vi "HEWH Mixing Valve.vi"(8 "Error In":errorcluster, 9 "Disable ERD (Main)":bool, 10 "ERD Data Out":T4[](array[typedef]) {"ERD Number" format="%.0x"}, 11 "ERD Data":T1 {"ERD Therm Data"."EEV Possition" format="%0.0f"; "ERD Therm Data"."T6" format="%.1f"; "ERD Therm Data"."T2" format="%.1f"; "ERD Therm Data"."T3a" format="%.1f"; "ERD Therm Data"."T3b" format="%.1f"; "ERD Therm Data"."T4" format="%.1f"; "ERD Therm Data"."T5" format="%.1f"; "ERD Therm Data"."Current" format="%.1f"}) -> (0 "Error Out":errorcluster, 3 "ERD Data Out":T1 {"ERD Therm Data"."EEV Possition" format="%0.0f"; "ERD Therm Data"."T6" format="%.1f"; "ERD Therm Data"."T2" format="%.1f"; "ERD Therm Data"."T3a" format="%.1f"; "ERD Therm Data"."T3b" format="%.1f"; "ERD Therm Data"."T4" format="%.1f"; "ERD Therm Data"."T5" format="%.1f"; "ERD Therm Data"."Current" format="%.1f"})   [LabVIEW 2016]
uses:
  type defs/ERD Read Data Out.ctl
  type defs/HEWH ERD Data.ctl
  type defs/HEWH Faults.ctl
  type defs/HEWH Mixing Valve.ctl
  library/GEA2_Toolkit.lvlib
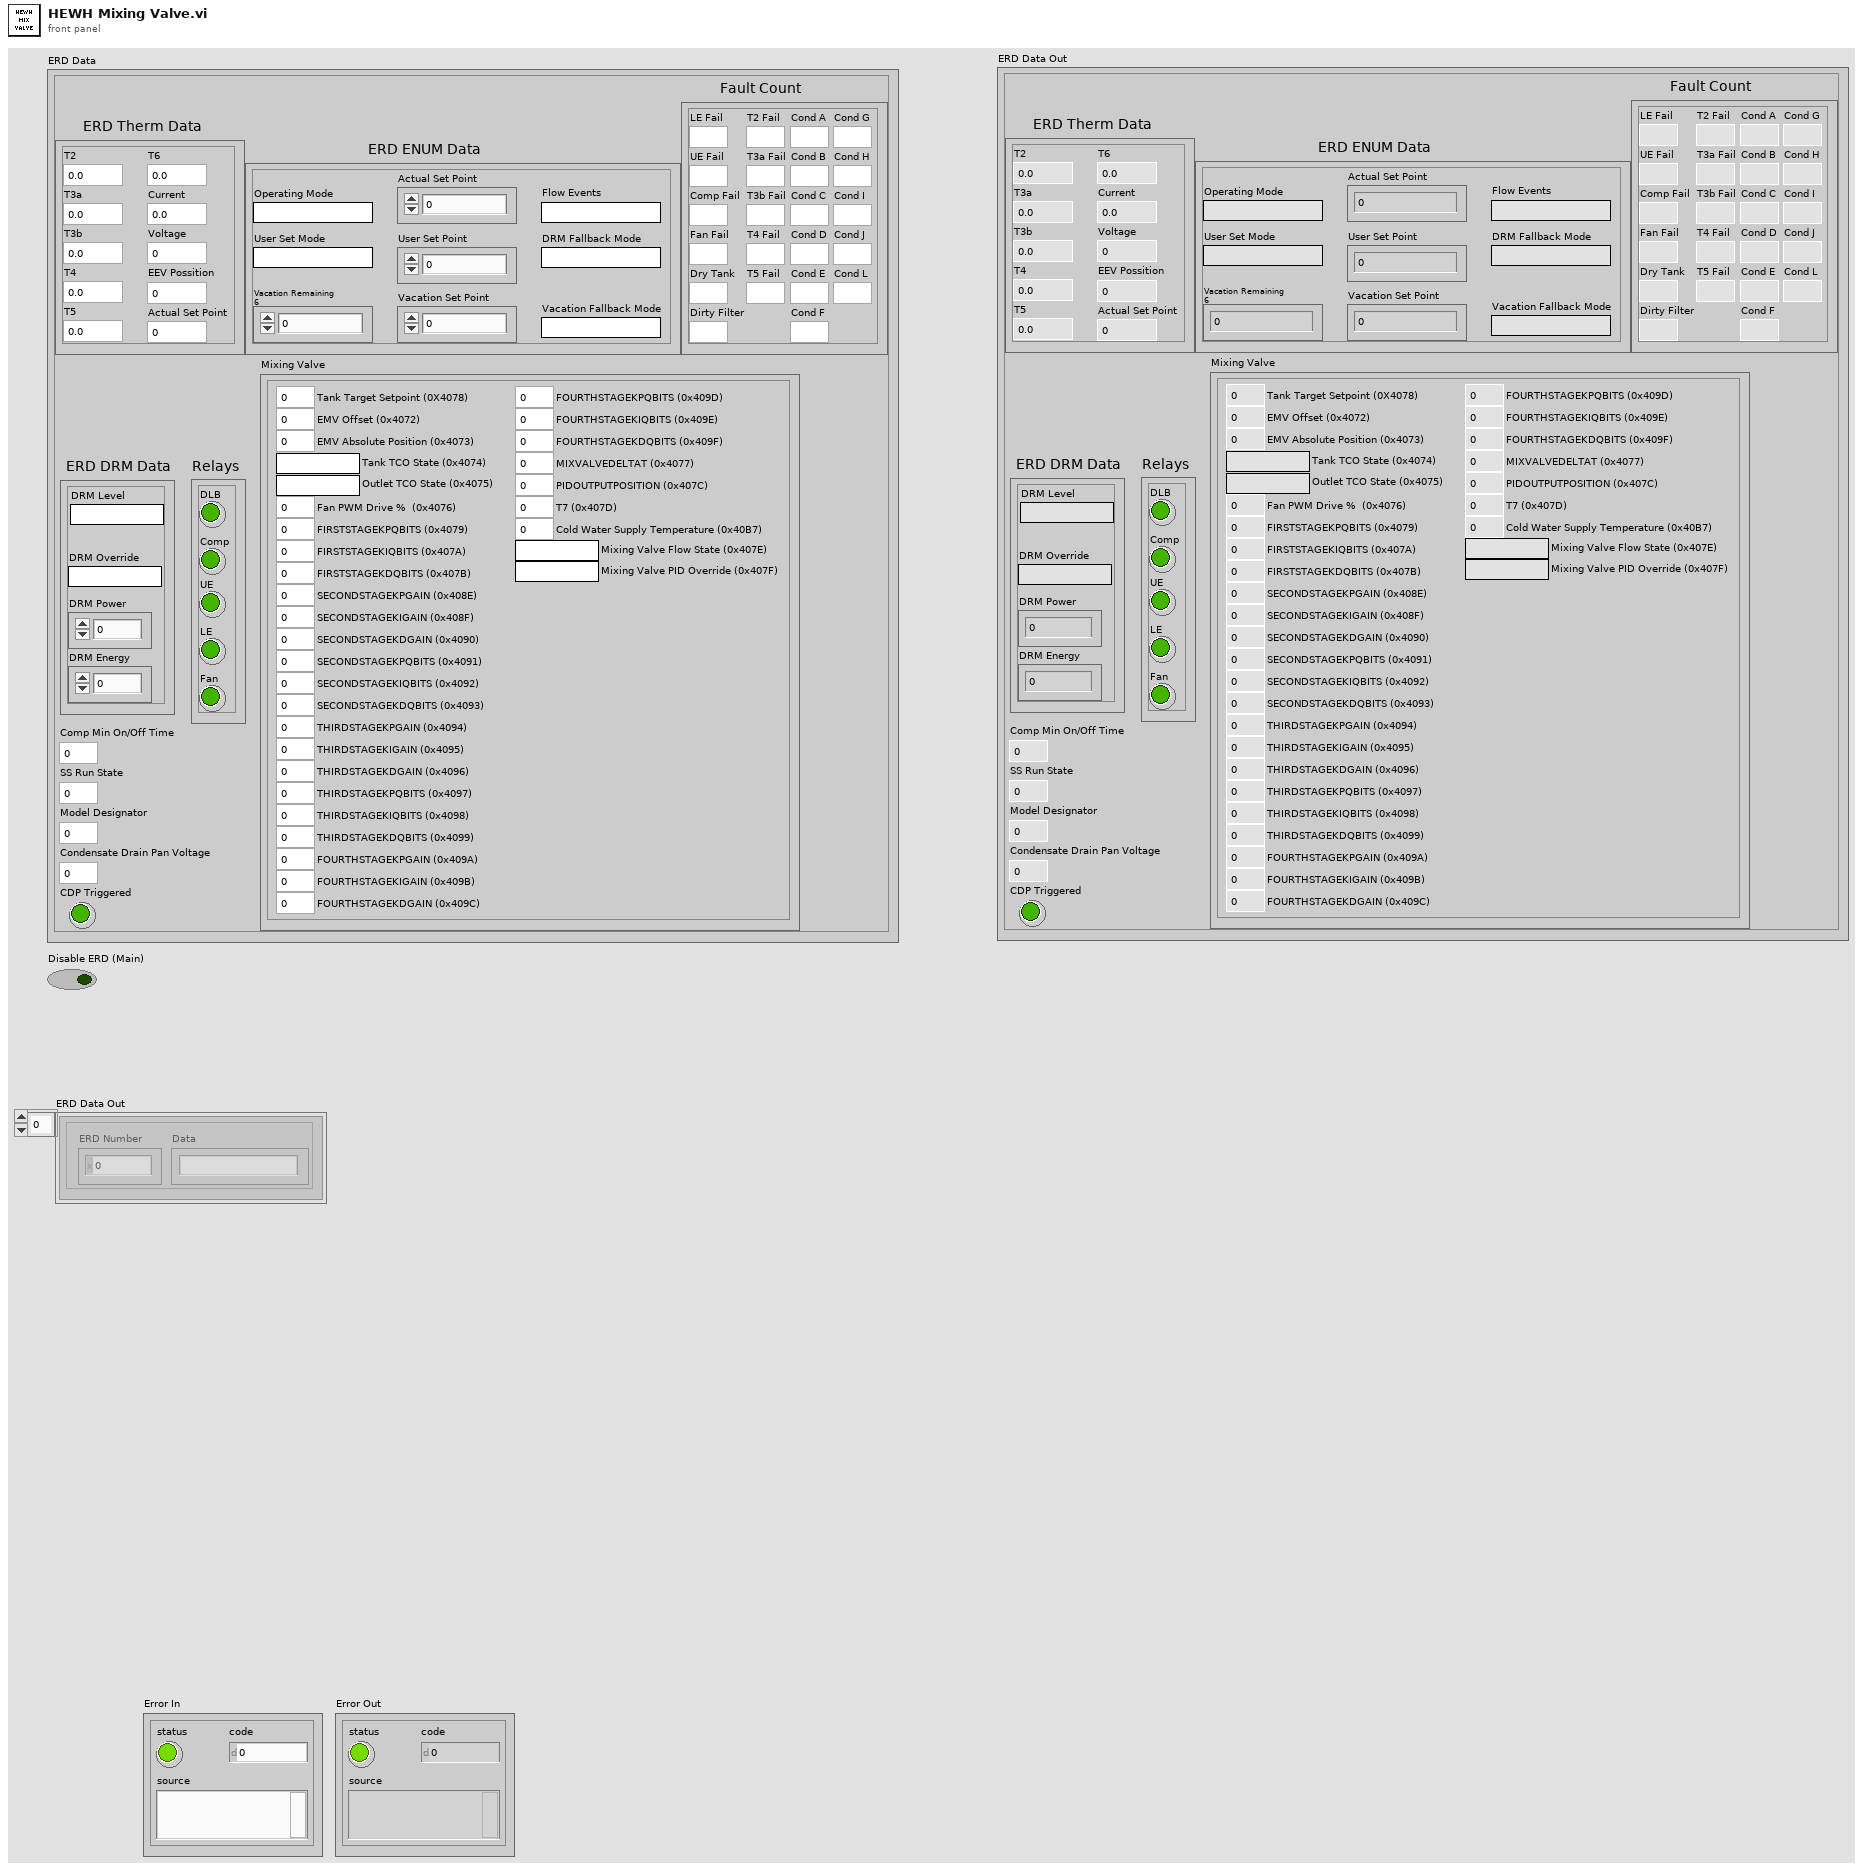
[diagram p1: front panel]
types:
  T1 = typedef "HEWH ERD Data.ctl" = cluster{"ERD Therm Data":cluster{"T2":dbl, "T3a":dbl, "T3b":dbl, "T4":dbl, "T5":dbl, "T6":dbl, "Current":dbl, "Voltage":dbl, "EEV Possition":dbl, "Actual Set Point":dbl}, "ERD ENUM Data":cluster{"Actual Set Point":dbl, "Flow Events":string, "User Set Mode":string, "Operating Mode":string, "DRM Fallback Mode":string, "Vacation Fallback Mode":string, "User Set Point":dbl, "Vacation Set Point":dbl, "Vacation Remaining\n6":dbl}, "ERD DRM Data":cluster{"DRM Level":string, "DRM Override":string, "DRM Power":dbl, "DRM Energy":dbl}, "Fault Count":T2, "Relays":cluster{"DLB":bool, "Comp":bool, "UE":bool, "LE":bool, "Fan":bool}, "Comp Min On/Off Time":u16, "SS Run State":u16, "Condensate Drain Pan Voltage":u16, "CDP Triggered":bool, "Model Designator":u8, "Mixing Valve":T3}
  T2 = typedef "HEWH Faults.ctl" = cluster{"LE Fail":u32, "UE Fail":u32, "Comp Fail":u32, "T2 Fail":u32, "T3a Fail":u32, "T3b Fail":u32, "T4 Fail":u32, "T5 Fail":u32, "Cond A":u32, "Cond B":u32, "Cond C":u32, "Cond D":u32, "Cond E":u32, "Cond F":u32, "Cond G":u32, "Cond H":u32, "Cond I":u32, "Cond J":u32, "Cond L":u32, "Fan Fail":u32, "Dirty Filter":u32, "Dry Tank":u32}
  T3 = typedef "HEWH Mixing Valve.ctl" = cluster{"Tank Target Setpoint (0X4078)":dbl, "EMV Offset (0x4072)":dbl, "EMV Absolute Position (0x4073)":dbl, "Tank TCO State (0x4074)":string, "Outlet TCO State (0x4075)":string, "Fan PWM Drive %  (0x4076)":dbl, "FIRSTSTAGEKPQBITS (0x4079)":dbl, "FIRSTSTAGEKIQBITS (0x407A)":dbl, "FIRSTSTAGEKDQBITS (0x407B)":dbl, "SECONDSTAGEKPGAIN (0x408E)":dbl, "SECONDSTAGEKIGAIN (0x408F)":dbl, "SECONDSTAGEKDGAIN (0x4090)":dbl, "SECONDSTAGEKPQBITS (0x4091)":dbl, "SECONDSTAGEKIQBITS (0x4092)":dbl, "SECONDSTAGEKDQBITS (0x4093)":dbl, "THIRDSTAGEKPGAIN (0x4094)":dbl, "THIRDSTAGEKIGAIN (0x4095)":dbl, "THIRDSTAGEKDGAIN (0x4096)":dbl, "THIRDSTAGEKPQBITS (0x4097)":dbl, "THIRDSTAGEKIQBITS (0x4098)":dbl, "THIRDSTAGEKDQBITS (0x4099)":dbl, "FOURTHSTAGEKPGAIN (0x409A)":dbl, "FOURTHSTAGEKIGAIN (0x409B)":dbl, "FOURTHSTAGEKDGAIN (0x409C)":dbl, "FOURTHSTAGEKPQBITS (0x409D)":dbl, "FOURTHSTAGEKIQBITS (0x409E)":dbl, "FOURTHSTAGEKDQBITS (0x409F)":dbl, "MIXVALVEDELTAT (0x4077)":dbl, "PIDOUTPUTPOSITION (0x407C)":dbl, "T7 (0x407D)":dbl, "Cold Water Supply Temperature (0x40B7)":dbl, "Mixing Valve Flow State (0x407E)":string, "Mixing Valve PID Override (0x407F)":string}
  T4 = typedef "GEA2_Toolkit.lvlib/ERD Read Data Out.ctl" = cluster{"ERD Number":u16, "Data":string}
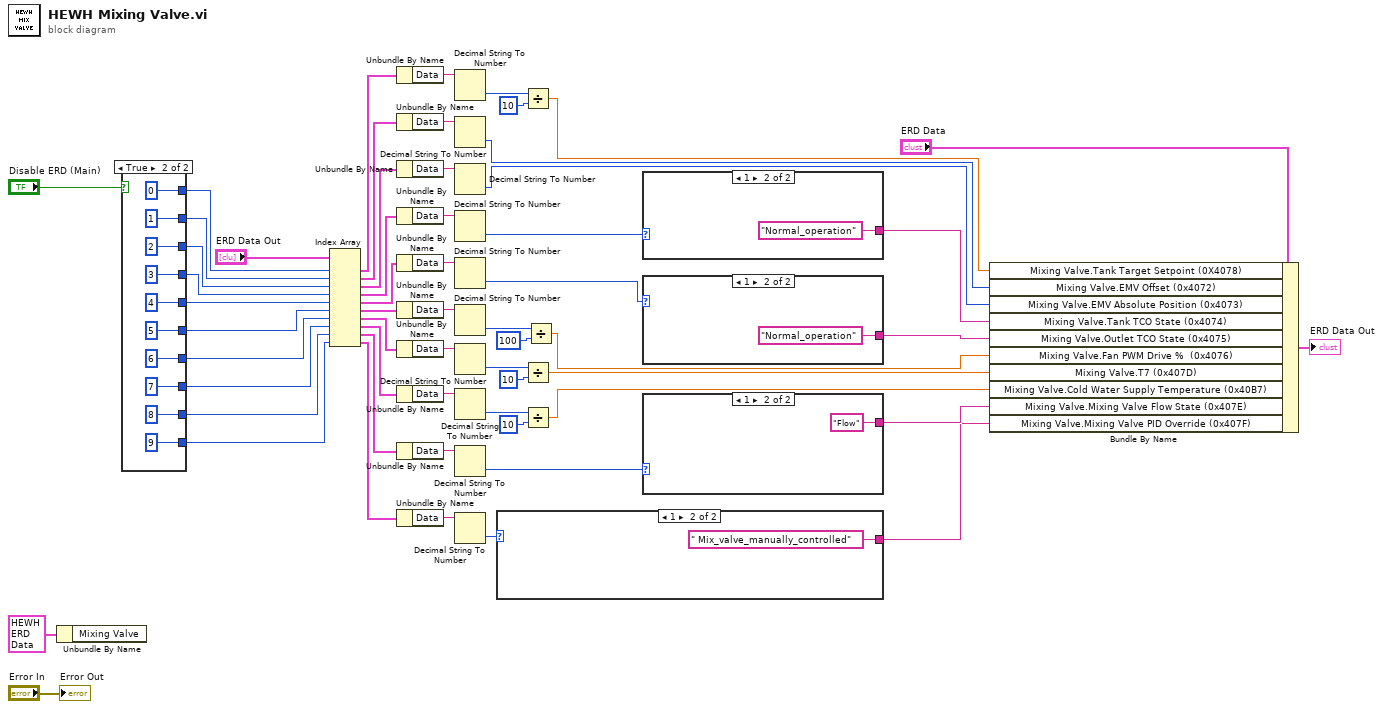
[diagram p0: block diagram]
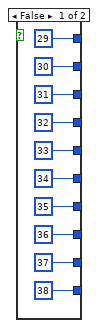
[diagram p2: hidden frame]
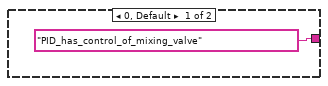
[diagram p3: hidden frame]
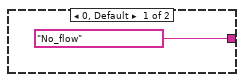
[diagram p4: hidden frame]
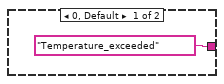
[diagram p5: hidden frame]
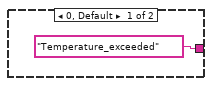
[diagram p6: hidden frame]
diagram:
  n1 = Unbundle By Name(T1 {"ERD Therm Data"={"T2"=0.0, "T3a"=0.0, "T3b"=0.0, "T4"=0.0, "T5"=0.0, "T6"=0.0, "Current"=0.0, "Voltage"=0.0, "EEV Possition"=0.0, "Actual Set Point"=0.0}, "ERD ENUM Data"={"Actual Set Point"=0.0, "Flow Events"="", "User Set Mode"="", "Operating Mode"="", "DRM Fallback Mode"="", "Vacation Fallback Mode"="", "User Set Point"=0.0, "Vacation Set Point"=0.0, "Vacation Remaining\n6"=0.0}, "ERD DRM Data"={"DRM Level"="", "DRM Override"="", "DRM Power"=0.0, "DRM Energy"=0.0}, "Fault Count"={"LE Fail"=0, "UE Fail"=0, "Comp Fail"=0, "T2 Fail"=0, "T3a Fail"=0, "T3b Fail"=0, "T4 Fail"=0, "T5 Fail"=0, "Cond A"=0, "Cond B"=0, "Cond C"=0, "Cond D"=0, "Cond E"=0, "Cond F"=0, "Cond G"=0, "Cond H"=0, "Cond I"=0, "Cond J"=0, "Cond L"=0, "Fan Fail"=0, "Dirty Filter"=0, "Dry Tank"=0}, "Relays"={"DLB"=FALSE, "Comp"=FALSE, "UE"=FALSE, "LE"=FALSE, "Fan"=FALSE}, "Comp Min On/Off Time"=0, "SS Run State"=0, "Condensate Drain Pan Voltage"=0, "CDP Triggered"=FALSE, "Model Designator"=0, "Mixing Valve"={"Tank Target Setpoint (0X4078)"=0.0, "EMV Offset (0x4072)"=0.0, "EMV Absolute Position (0x4073)"=0.0, "Tank TCO State (0x4074)"="", "Outlet TCO State (0x4075)"="", "Fan PWM Drive %  (0x4076)"=0.0, "FIRSTSTAGEKPQBITS (0x4079)"=0.0, "FIRSTSTAGEKIQBITS (0x407A)"=0.0, "FIRSTSTAGEKDQBITS (0x407B)"=0.0, "SECONDSTAGEKPGAIN (0x408E)"=0.0, "SECONDSTAGEKIGAIN (0x408F)"=0.0, "SECONDSTAGEKDGAIN (0x4090)"=0.0, "SECONDSTAGEKPQBITS (0x4091)"=0.0, "SECONDSTAGEKIQBITS (0x4092)"=0.0, "SECONDSTAGEKDQBITS (0x4093)"=0.0, "THIRDSTAGEKPGAIN (0x4094)"=0.0, "THIRDSTAGEKIGAIN (0x4095)"=0.0, "THIRDSTAGEKDGAIN (0x4096)"=0.0, "THIRDSTAGEKPQBITS (0x4097)"=0.0, "THIRDSTAGEKIQBITS (0x4098)"=0.0, "THIRDSTAGEKDQBITS (0x4099)"=0.0, "FOURTHSTAGEKPGAIN (0x409A)"=0.0, "FOURTHSTAGEKIGAIN (0x409B)"=0.0, "FOURTHSTAGEKDGAIN (0x409C)"=0.0, "FOURTHSTAGEKPQBITS (0x409D)"=0.0, "FOURTHSTAGEKIQBITS (0x409E)"=0.0, "FOURTHSTAGEKDQBITS (0x409F)"=0.0, "MIXVALVEDELTAT (0x4077)"=0.0, "PIDOUTPUTPOSITION (0x407C)"=0.0, "T7 (0x407D)"=0.0, "Cold Water Supply Temperature (0x40B7)"=0.0, "Mixing Valve Flow State (0x407E)"="", "Mixing Valve PID Override (0x407F)"=""}} ("ERD Data")) -> ()  [unwired: 1 out]
  n2 = case shown="True" "Disable ERD (Main)" {
    tunnel: [29 ("index") 0 ("index")] -> w56
    tunnel: [30 ("index") 1 ("index")] -> w41
    tunnel: [31 ("index") 2 ("index")] -> w40
    tunnel: [32 ("index") 3 ("index")] -> w39
    tunnel: [33 ("index") 4 ("index")] -> w38
    tunnel: [34 ("index") 5 ("index")] -> w37
    tunnel: [35 ("index") 6 ("index")] -> w36
    tunnel: [36 ("index") 7 ("index")] -> w35
    tunnel: [37 ("index") 8 ("index")] -> w34
    tunnel: [38 ("index") 9 ("index")] -> w33
    frame False {
    }
    frame True {
    }
  }
  n3 = Index Array(array="ERD Data Out", index #1=w56, index #2=w41, index #3=w40, index #4=w39, index #5=w38, index #6=w37, index #7=w36, index #8=w35, index #9=w34, index #10=w33) -> (element #1=w55:T4, element #2=w48:T4, element #3=w46:T4, element #4=w44:T4, element #5=w43:T4, element #6=w42:T4, element #7=w8:T4, element #8=w7:T4, element #9=w6:T4, element #10=w5:T4)
  n4 = Unbundle By Name(w55) -> ("Data"=w54:string)
  n5 = Unbundle By Name(w48) -> ("Data"=w53:string)
  n6 = Unbundle By Name(w46) -> ("Data"=w52:string)
  n7 = Unbundle By Name(w44) -> ("Data"=w51:string)
  n8 = Unbundle By Name(w43) -> ("Data"=w50:string)
  n9 = Unbundle By Name(w42) -> ("Data"=w49:string)
  n10 = Unbundle By Name(w8) -> ("Data"=w32:string)
  n11 = Unbundle By Name(w7) -> ("Data"=w23:string)
  n12 = Unbundle By Name(w6) -> ("Data"=w14:string)
  n13 = Unbundle By Name(w5) -> ("Data"=w13:string)
  n14 = Decimal String To Number(string=w54) -> (number=w31:i32)  [unwired: 2 in, 1 out]
  n15 = Decimal String To Number(string=w53) -> (number=w47:i32)  [unwired: 2 in, 1 out]
  n16 = Decimal String To Number(string=w52) -> (number=w45:i32)  [unwired: 2 in, 1 out]
  n17 = Decimal String To Number(string=w51) -> (number=w21:i32)  [unwired: 2 in, 1 out]
  n18 = Decimal String To Number(string=w50) -> (number=w19:i32)  [unwired: 2 in, 1 out]
  n19 = Decimal String To Number(string=w49) -> (number=w17:i32)  [unwired: 2 in, 1 out]
  n20 = Decimal String To Number(string=w32) -> (number=w27:i32)  [unwired: 2 in, 1 out]
  n21 = Decimal String To Number(string=w23) -> (number=w24:i32)  [unwired: 2 in, 1 out]
  n22 = Decimal String To Number(string=w14) -> (number=w11:i32)  [unwired: 2 in, 1 out]
  n23 = Decimal String To Number(string=w13) -> (number=w9:i32)  [unwired: 2 in, 1 out]
  n24 = case shown="1" w9 {
    tunnel: ["PID_has_control_of_mixing_valve" " Mix_valve_manually_controlled"] -> w10
    frame 0, Default {
    }
    frame 1 {
    }
  }
  n25 = Divide(x=w31, y=10) -> (x/y=w29:dbl)
  n26 = Divide(x=w27, y=10) -> (x/y=w26:dbl)
  n27 = Divide(x=w24, y=10) -> (x/y=w22:dbl)
  n28 = Divide(x=w17, y=100) -> (x/y=w15:dbl)
  n29 = case shown="1" w21 {
    tunnel: ["Temperature_exceeded" "Normal_operation"] -> w20
    frame 0, Default {
    }
    frame 1 {
    }
  }
  n30 = case shown="1" w19 {
    tunnel: ["Temperature_exceeded" "Normal_operation"] -> w18
    frame 0, Default {
    }
    frame 1 {
    }
  }
  n31 = case shown="1" w11 {
    tunnel: ["No_flow" "Flow"] -> w12
    frame 0, Default {
    }
    frame 1 {
    }
  }
  n32 = Bundle By Name(cluster="ERD Data", "Mixing Valve.Tank Target Setpoint (0X4078)"=w29, "Mixing Valve.EMV Offset (0x4072)"=w47, "Mixing Valve.EMV Absolute Position (0x4073)"=w45, "Mixing Valve.Tank TCO State (0x4074)"=w20, "Mixing Valve.Outlet TCO State (0x4075)"=w18, "Mixing Valve.Fan PWM Drive %  (0x4076)"=w15, "Mixing Valve.T7 (0x407D)"=w26, "Mixing Valve.Cold Water Supply Temperature (0x40B7)"=w22, "Mixing Valve.Mixing Valve Flow State (0x407E)"=w12, "Mixing Valve.Mixing Valve PID Override (0x407F)"=w10) -> (→"ERD Data Out":T1)
  "Error Out" <- "Error In"
